vi "Options.vi"(8 "error in (no error)":errorcluster) -> (0 "error out":errorcluster)   [LabVIEW 2017]
uses:
  <vilib>/registry/registry.llb/Registry RtKey.ctl
  <vilib>/registry/registry.llb/Registry SAM.ctl
  <vilib>/registry/registry.llb/Write Registry Value Simple STR.vi
panel:
  in  "Touch":bool
  out "Network Configuration Label":string
  in  "IP Address":string
  in  "Apply":bool
  # "Configuration"
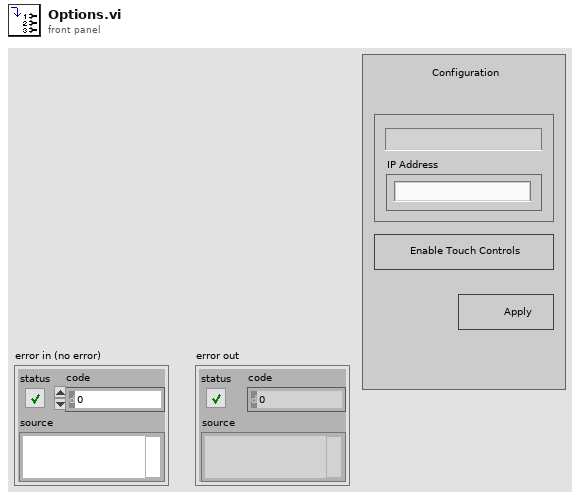
[diagram p1: front panel]
types:
  T1 = enum32{"REG_OPTION_NON_VOLATILE", "REG_OPTION_VOLATILE", "REG_OPTION_BACKUP_RESTORE"}
  T2 = typedef "Registry SAM.ctl" = enum32{"KEY_QUERY_VALUE", "KEY_SET_VALUE", "KEY_CREATE_SUB_KEY", "KEY_ENUMERATE_SUB_KEYS", "KEY_NOTIFY", "KEY_CREATE_LINK", "KEY_READ", "KEY_WRITE", "KEY_ALL_ACCESS", "KEY_READ | KEY_WRITE"}
  T3 = typedef "Registry RtKey.ctl" = enum32{"HKEY_CLASSES_ROOT", "HKEY_CURRENT_USER", "HKEY_LOCAL_MACHINE", "HKEY_USERS", "HKEY_PERFORMANCE_DATA", "HKEY_CURRENT_CONFIG", "HKEY_DYN_DATA"}
  T4 = typedef "Registry refnum.ctl" = refnum<k1>
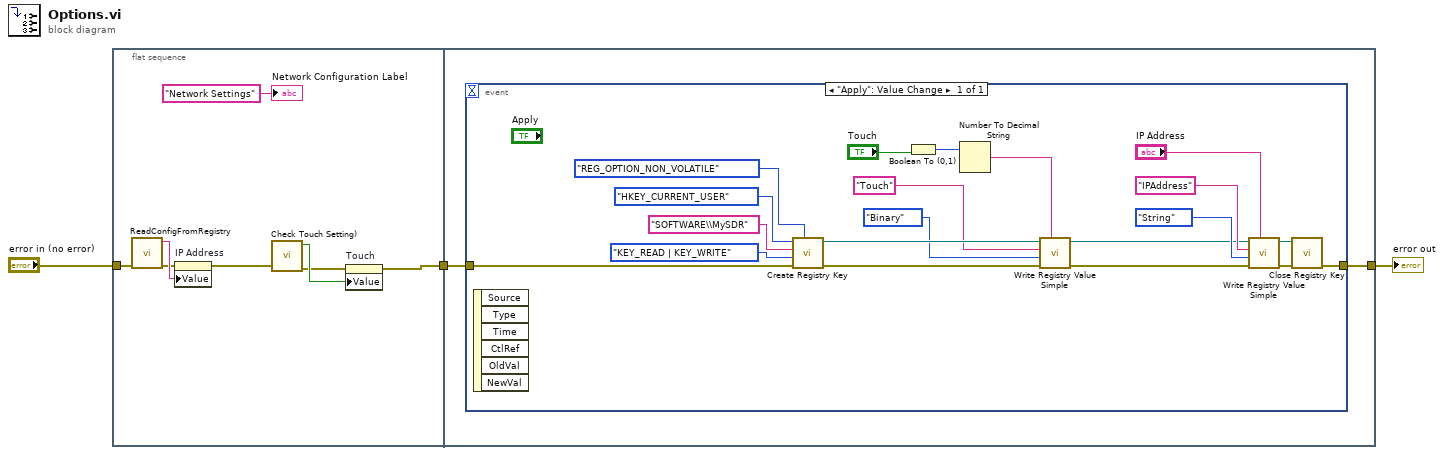
[diagram p0: block diagram]
diagram:
  n1 = flat-sequence {
    tunnel: "error in (no error)" -> [w8]
    tunnel: [w4] -> w2
    tunnel: w2 -> [w13]
    tunnel: [w12] -> w1
    frame #0 {
      n2 = call "ReadConfigFromRegistry.vi"("error in (no error)"=w8) -> ("error out"=w9:errorcluster, "String/Binary data"=w10:string)  [unwired: 9 in]
      n3 = property on="IP Address" class="Str"(error in=w9, "Value"=w10) -> (error out=w7:errorcluster)  [unwired: 1 in, 1 out]
      n4 = call "Check Touch Setting).vi"("error in (no error)"=w7) -> ("error out"=w5:errorcluster, "Boolean"=w6:bool)  [unwired: 9 in]
      n5 = property on="Touch" class="Bool (strict)"(error in=w5, "Value"=w6) -> (error out=w4:errorcluster)  [unwired: 1 in, 1 out]
      "Network Configuration Label" <- "Network Settings" ("Network Configuration Label")
    }
    frame #1 {
      n6 = event shown="[0] \"Apply\": Value Change" {
        selector: _ -> [_]
        dyn-events: _ -> [_]
        timeout: _ -> [_]
        tunnel: w13 -> [w25]
        tunnel: [w24] -> w12
        event "Apply": Value Change {
          n7 = event-data() -> ()  [unwired: 1 in, 6 out]
          n8 = call <vilib>:"Create Registry Key.vi"("options"=T1."REG_OPTION_NON_VOLATILE", "error in (no error)"=w25, "security access mask (KEY_READ | KEY_WRITE)"=Registry_SAM."KEY_READ | KEY_WRITE", "subkey"="SOFTWARE\\MySDR", "root key (HKEY_LOCAL_MACHINE)"=Registry_RtKey."HKEY_CURRENT_USER") -> ("error out"=w22:errorcluster, "refnum out"=w21:T4)  [unwired: 4 in, 1 out]
          n9 = Boolean To (0,1)(Boolean="Touch") -> (0, 1=w17:i16)
          n10 = Number To Decimal String(number=w17) -> (decimal integer string=w15:string)  [unwired: 1 in]
          n11 = call-poly <vilib>:"Write Registry Value Simple.vi"("String/Binary data"=w15, "error in (no error)"=w22, "simple data type"=enum16{"String", "Binary", "DWORD"}."Binary", "value"="Touch", "refnum"=w21) -> ("error out"=w19:errorcluster, "refnum out"=w18:T4)  [unwired: 3 in]
          n12 = call-poly <vilib>:"Write Registry Value Simple.vi"("String/Binary data"="IP Address", "error in (no error)"=w19, "simple data type"=enum16{"String", "Binary", "DWORD"}."String", "value"="IPAddress", "refnum"=w18) -> ("error out"=w28:errorcluster, "refnum out"=w27:T4)  [unwired: 3 in]
          n13 = call <vilib>:"Close Registry Key.vi"("error in (no error)"=w28, "refnum"=w27) -> ("error out"=w24:errorcluster)  [unwired: 5 in]
        }
      }
    }
  }
  "error out" <- w1
